vi "GetTerms.vi"(0 "XRef":T12, 1 "State In":T10) -> (14 "Terms":T2, 15 "Fatal Error Out":T1)   [LabVIEW 2018, in "RetryNode.xnode"]
uses:
  RetryNode.xnode
  <vilib>/XNodeSupport/XNodeXNodeRef.ctl
  State.ctl
  <vilib>/Utility/miscctls.llb/LVRectTypeDef.ctl
  <vilib>/XNodeSupport/XNodeTerm4Array.ctl
  <vilib>/XNodeSupport/XNodeTerm4.ctl
  <vilib>/XNodeSupport/XNodeString.ctl
  <vilib>/XNodeSupport/XNodeVariant.ctl
  <vilib>/XNodeSupport/XNodeRect32.ctl
  <vilib>/XNodeSupport/XNodeInt.ctl
  <vilib>/XNodeSupport/XNodeBool.ctl
  <vilib>/XNodeSupport/XNodeTermDirection.ctl
  <vilib>/XNodeSupport/XNodeErrorCluster.ctl
  <vilib>/XNodeSupport/NI_XNodeSupport.lvlib
panel:
  out "Width":u32
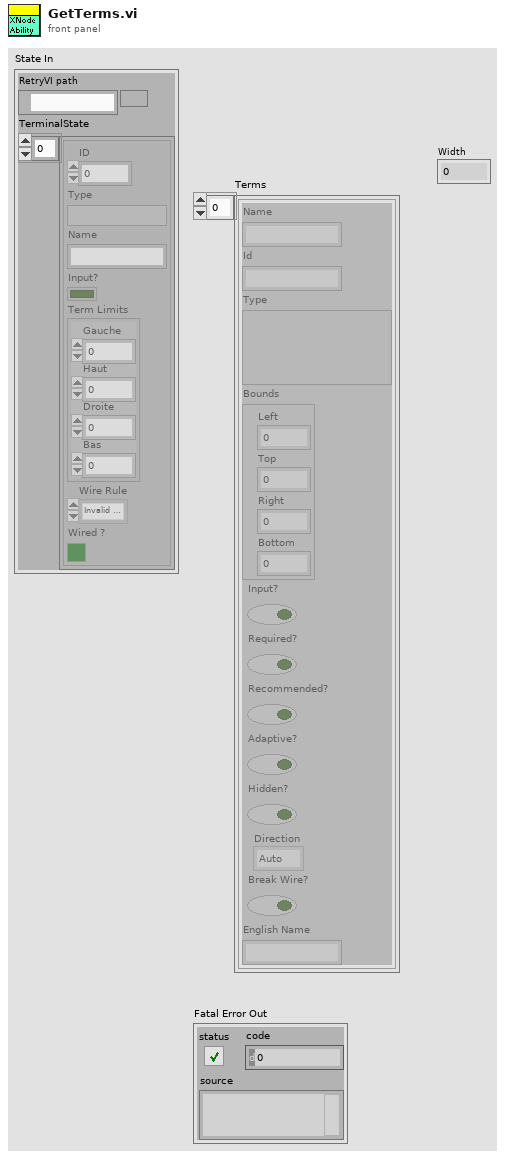
[diagram p1: front panel]
types:
  T1 = typedef "NI_XNodeSupport.lvlib/XNodeErrorCluster.ctl" = errorcluster
  T2 = typedef "NI_XNodeSupport.lvlib/XNodeTerm4Array.ctl" = T3[]
  T3 = typedef "NI_XNodeSupport.lvlib/XNodeTerm4.ctl" = cluster{"Name":T4, "Id":T4, "Type":T5, "Bounds":T6, "Input?":T8, "Required?":T8, "Recommended?":T8, "Adaptive?":T8, "Hidden?":T8, "Direction":T9, "Break Wire?":T8, "English Name":T4}
  T4 = typedef "NI_XNodeSupport.lvlib/XNodeString.ctl" = string
  T5 = typedef "NI_XNodeSupport.lvlib/XNodeVariant.ctl" = variant
  T6 = typedef "NI_XNodeSupport.lvlib/XNodeRect32.ctl" = cluster{"Left":T7, "Top":T7, "Right":T7, "Bottom":T7}
  T7 = typedef "NI_XNodeSupport.lvlib/XNodeInt.ctl" = i32
  T8 = typedef "NI_XNodeSupport.lvlib/XNodeBool.ctl" = bool
  T9 = typedef "NI_XNodeSupport.lvlib/XNodeTermDirection.ctl" = enum32{"Auto", "Up", "Down", "Left", "Right", "Center"}
  T10 = typedef "RetryNode.xnode/State.ctl" = cluster{"RetryVI path":path, "TerminalState":cluster{"ID":i32, "Type":variant, "Name":string, "Input?":bool, "Term Limits":T11, "Wire Rule":enum16{"Invalid Wire Rule", "Required", "Recommended", "Optional", "Dynamic Dispatch"}, "Wired ?":bool}[]}
  T11 = typedef "LVRectTypeDef.ctl" = cluster{"Left":i16, "Top":i16, "Right":i16, "Bottom":i16}
  T12 = typedef "NI_XNodeSupport.lvlib/XNodeXNodeRef.ctl" = refnum<vi>
  T13 = typedef "LVBoundsTypeDef.ctl" = cluster{"Width":u32, "Height":u32}
  T14 = cluster{"ID":i32, "Type":variant, "Name":string, "Input?":bool, "Term Limits":T11, "Wire Rule":enum16{"Invalid Wire Rule", "Required", "Recommended", "Optional", "Dynamic Dispatch"}, "Wired ?":bool}[]
  T15 = enum16{"Invalid Wire Rule", "Required", "Recommended", "Optional", "Dynamic Dispatch"}
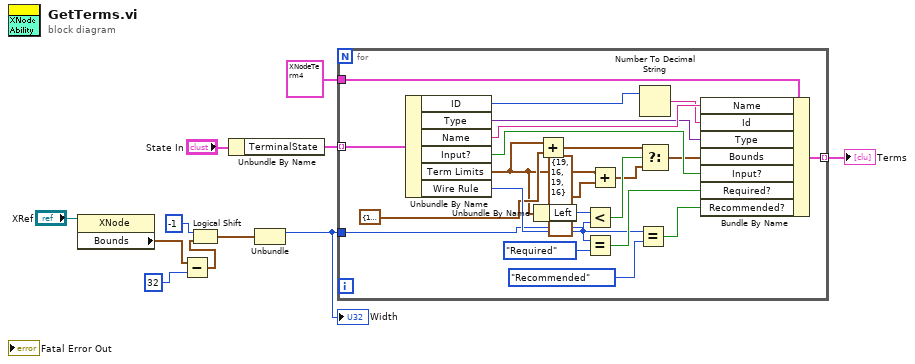
[diagram p0: block diagram]
diagram:
  n1 = property class="XNode"(reference="XRef") -> ("Bounds"=w3:T13)  [unwired: 1 in, 2 out]
  n2 = Subtract(x=w3, y=i16 32) -> (x-y=w1:T13)
  n3 = Logical Shift(y=i16 -1, x=w1) -> (x << y=w5:T13)
  n4 = Unbundle By Name("State In") -> ("TerminalState"=w11:T14)
  n5 = Unbundle(w5) -> ("Width"=w4:u32)  [unwired: 1 out]
  "Width" <- w4
  n6 = for {
    tunnel: w11 -> [w33] mode=indexing
    tunnel: T3 {"Name"="", "Id"="", "Type"=variant, "Bounds"={"Left"=0, "Top"=0, "Right"=0, "Bottom"=0}, "Input?"=FALSE, "Required?"=FALSE, "Recommended?"=FALSE, "Adaptive?"=FALSE, "Hidden?"=FALSE, "Direction"=enum."Auto", "Break Wire?"=FALSE, "English Name"=""} ("Term 4") -> [w32]
    tunnel: [w25] -> w8 mode=indexing
    tunnel: w4 -> [w20]
    n7 = Unbundle By Name(w33) -> ("ID"=w30:i32, "Type"=w28:variant, "Name"=w31:string, "Input?"=w27:bool, "Term Limits"=w13:T11, "Wire Rule"=w23:T15)
    n8 = Unbundle By Name(w13) -> ("Left"=w19:i16)
    n9 = Add(x=w13, y=cluster{i32, i32, i32, i32} {13, 16, 13, 16}) -> (x+y=w16:cluster{i32, i32, i32, i32})
    n10 = Less?(x=w19, y=w20) -> (x < y?=w18:bool)
    n11 = Equal?(x=w23, y=T15."Required") -> (x = y?=w26:bool)
    n12 = Add(x=w13, y=cluster{i32, i32, i32, i32} {19, 16, 19, 16}) -> (x+y=w12:cluster{i32, i32, i32, i32})
    n13 = Equal?(x=w23, y=T15."Recommended") -> (x = y?=w21:bool)
    n14 = Number To Decimal String(number=w30) -> (decimal integer string=w29:string)  [unwired: 1 in]
    n15 = Select(t=w16, s=w18, f=w12) -> (s? t:f=w17:cluster{i32, i32, i32, i32})
    n16 = Bundle By Name(cluster=w32, "Name"=w31, "Id"=w29, "Type"=w28, "Bounds"=w17, "Input?"=w27, "Required?"=w26, "Recommended?"=w21) -> (w25:T3)
  }
  "Terms" <- w8
